vi "RC_STM_Client 1.vi"() -> ()   [LabVIEW 2019, in "RemoteControl.STM.lvclass"]
uses:
  RemoteControl.STM.lvclass
  RemoteControl/RemoteControl.lvclass
  <userlib>/_OpenG.lib/numeric/numeric.llb/Random Number Within Range - I32__ogtk.vi
  <userlib>/_OpenG.lib/error/error.llb/Filter Error Codes (Array)__ogtk.vi
  C:/user/patrick/git/LevyLab-Instrument-Framework/2019 instrument Folder/lvsrc/SMOs/RemoteControl/RemoteControl.lvclass
  C:/user/patrick/git/LevyLab-Instrument-Framework/2019 instrument Folder/lvsrc/SMOs/LevyLab/LevyLab.lvclass
  C:/Program Files (x86)/National Instruments/LabVIEW 2019/vi.lib/JKI/JKI SMO/SMO/SMO.lvclass
panel:
  in  "Test RC Client":bool
  in  "milliseconds to wait":u32
  out "time (1 message) (ms)":u32
  out "startup time (ms)":u32
  out "messsages/s":dbl
  in  "remote port":u16=6341
  in  "address":string
  out "Data reponse":string
  out "Messages":i32
  in  "Stop":bool
  out "Command reponse":string
  out "Command":string
  out "meta data\n(available commands)":string
  out "error out":errorcluster
  # "CLIENT (API)"
  # "Connection info"
  # "Message Sent"
  # "Message Received"
  # "Metrics"
  # "1"
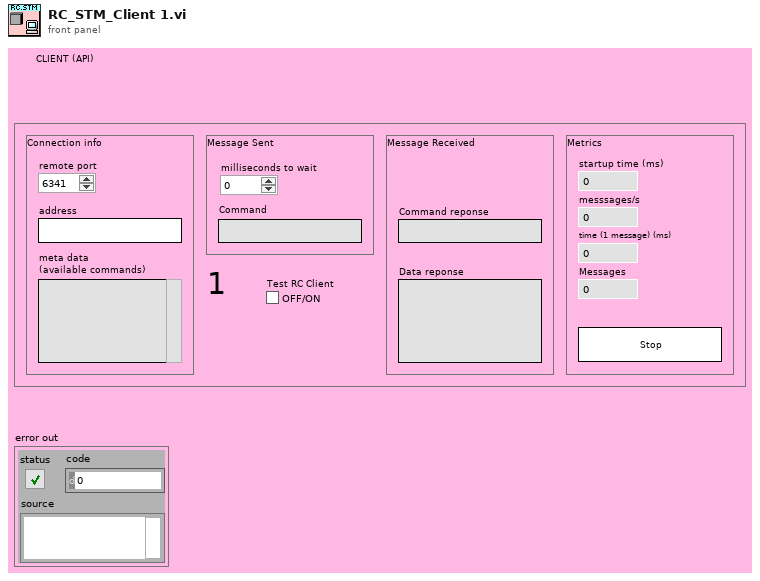
[diagram p1: front panel]
types:
  T1 = typedef "NI STM.lvlib/MetaDataElement.ctl" = string
  T2 = cluster{"Command out":string, "Data out":variant, i32}
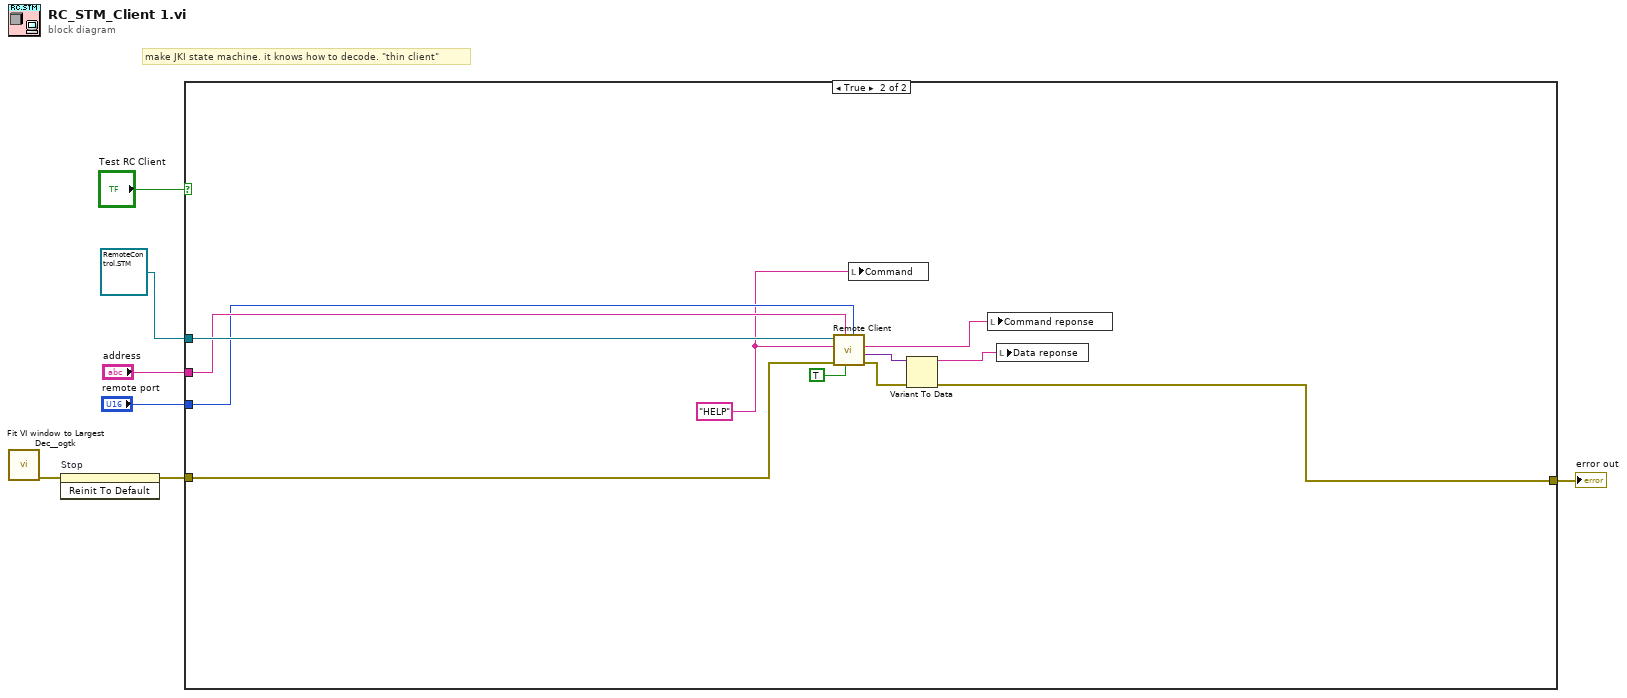
[diagram p0: block diagram]
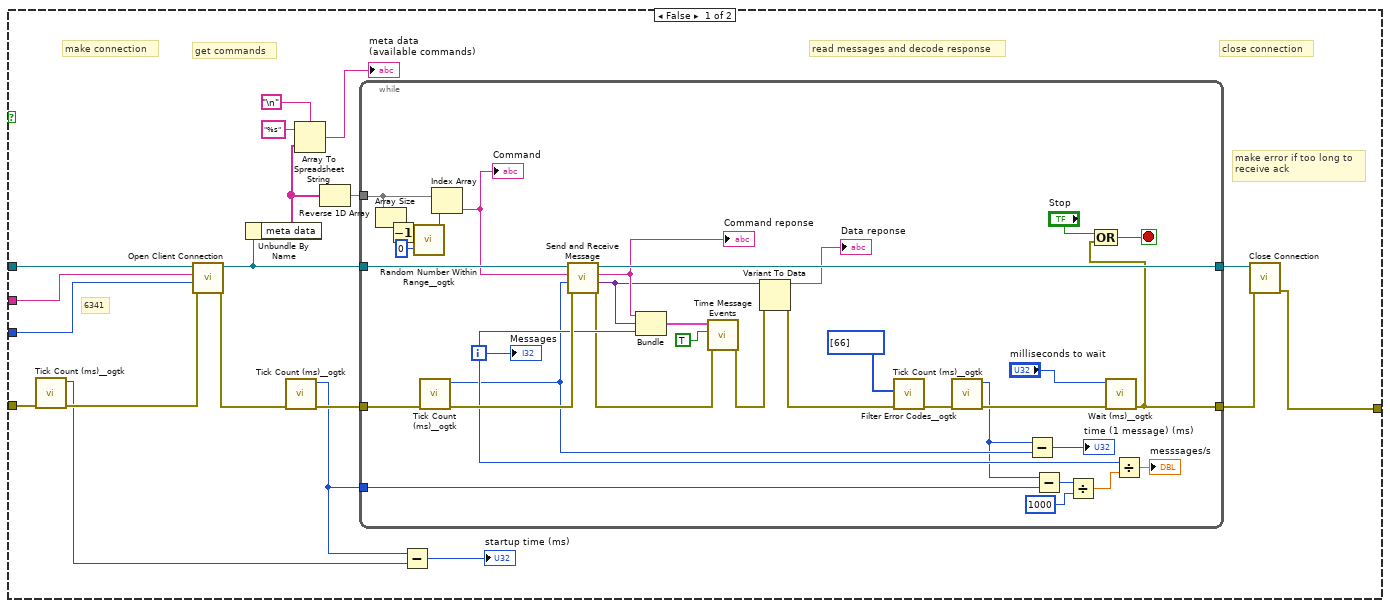
[diagram p2: hidden frame]
diagram:
  # "make JKI state machine. it knows how to decode. \"thin client\""
  n1 = call <userlib>:"Fit VI window to Largest Dec__ogtk.vi"() -> ("error out"=w2:errorcluster)  [unwired: 6 in, 1 out]
  n2 = invoke on="Stop" class="Bool" method="Reinit To Default"(error in=w2) -> (error out=w3:errorcluster)  [unwired: 2 in, 2 out]
  n3 = case shown="True" "Test RC Client" {
    tunnel: refnum<class "RemoteControl.STM.lvclass"> refnum ("RemoteControl.STM in") -> [w12 w71]
    tunnel: "remote port" -> [w11 w63]
    tunnel: "address" -> [w10 w64]
    tunnel: w3 -> [w9 w65]
    tunnel: [w8 w66] -> w1
    frame False {
      # "close connection"
      # "read messages and decode response"
      # "get commands"
      # "make connection"
      # "6341"
      # "make error if too long to\nreceive ack"
      n4 = call <userlib>:"Tick Count (ms)__ogtk.vi"("error in (no error)"=w9) -> ("error out"=w22:errorcluster, "millisecond timer value"=w18:u32)  [unwired: 9 in]
      n5 = call-dynamic "Open Client Connection.vi"("error in (no error)"=w22, "Port"=w11, "address"=w10, "RemoteControl.STM in"=w12) -> ("error out"=w21:errorcluster, "RemoteControl.STM out"=w24:refnum<class "RemoteControl.STM.lvclass">)  [unwired: 6 in]
      n6 = Unbundle By Name(w24) -> ("meta data"=w17:T1[])
      n7 = call <userlib>:"Tick Count (ms)__ogtk.vi"("error in (no error)"=w21) -> ("error out"=w20:errorcluster, "millisecond timer value"=w13:u32)  [unwired: 9 in]
      n8 = Array To Spreadsheet String(delimiter (Tab)="\n", array=w17, 3:"%s" ("format string")) -> (spreadsheet string=→"meta data\n(available commands)":string)
      n9 = Reverse 1D Array(array=w17) -> (reversed array=w23:T1[])
      n10 = while {
        tunnel: [w36] -> w26
        tunnel: [w57] -> w25
        tunnel: w20 -> [w52]
        tunnel: w24 -> [w58]
        tunnel: w23 -> [w40]
        tunnel: w13 -> [w27]
        i -> [w49]
        stop <- w60 stop-if-true
        n11 = Array Size(array=w40) -> (size(s)=w41:i32)
        n12 = Decrement(x=w41) -> (x-1=w39:i32)
        n13 = call-poly <userlib>:"Random Number Within Range__ogtk.vi"("High"=w39, "Low"=0) -> ("Random Number"=w43:i32)  [unwired: 3 in]
        n14 = call <userlib>:"Tick Count (ms)__ogtk.vi"("error in (no error)"=w52) -> ("error out"=w51:errorcluster, "millisecond timer value"=w37:u32)  [unwired: 9 in]
        n15 = Index Array(array=w40, index=w43) -> (element=w53:T1)
        "Command" <- w53
        n16 = call-dynamic "Send and Receive Message.vi"("error in (no error)"=w51, "Data"=w37, "Command"=w53, "RemoteControl in"=w58) -> ("error out"=w38:errorcluster, "Data out"=w35:variant, "Command out"=w50:string, "RemoteControl out"=w57:refnum<class "RemoteControl.STM.lvclass">)  [unwired: 4 in]
        "Command reponse" <- w50
        n17 = Bundle("Command out"=w50, "Data out"=w35, w49) -> (w48:T2)  [unwired: 1 in]
        n18 = call "Time Message Events.vi"("error in (no error)"=w38, "Debug Mode"=TRUE, "Message in"=w48) -> ("error out"=w34:errorcluster)  [unwired: 6 in, 2 out]
        n19 = Variant To Data(error in=w34, Variant=w35) -> (data=→"Data reponse":string, error out=w33:errorcluster)  [unwired: 1 in]
        n20 = call-poly <userlib>:"Filter Error Codes__ogtk.vi"("Error In"=w33, "Error Codes to Filter"=i32[] [66]) -> ("Error Out"=w56:errorcluster)  [unwired: 7 in, 2 out]
        n21 = call <userlib>:"Tick Count (ms)__ogtk.vi"("error in (no error)"=w56) -> ("error out"=w46:errorcluster, "millisecond timer value"=w29:u32)  [unwired: 9 in]
        n22 = Subtract(x=w29, y=w37) -> (x-y=→"time (1 message) (ms)":u32)
        n23 = Subtract(x=w29, y=w27) -> (x-y=w28:u32)
        n24 = Divide(x=w28, y=u32 1000) -> (x/y=w55:dbl)
        n25 = call <userlib>:"Wait (ms)__ogtk.vi"("error in (no error)"=w46, "milliseconds to wait"="milliseconds to wait") -> ("error out"=w36:errorcluster)  [unwired: 8 in, 1 out]
        n26 = Compound Arithmetic op=OR("Stop", w36) -> (w60:bool)
        n27 = Divide(x=w49, y=w55) -> (x/y=→"messsages/s":dbl)
        "Messages" <- w49
      }
      n28 = Subtract(x=w13, y=w18) -> (x-y=→"startup time (ms)":u32)
      n29 = call-dynamic "Close Connection.vi"("error in (no error)"=w26, "RemoteControl.STM in"=w25) -> ("error out"=w8:errorcluster)  [unwired: 8 in, 1 out]
    }
    frame True {
      w62 = "HELP" ("Command")
      n30 = call "Remote Client.vi"("Port"=w63, "Wait for Response?"=TRUE, "address"=w64, "error in (no error)"=w65, "Command"=w62, "RemoteControl in"=w71) -> ("error out"=w67:errorcluster, "Data out"=w70:variant, "Command out"=w69:string)  [unwired: 2 in, 1 out]
      n31 = local write "Command"(w62) -> ()
      n32 = Variant To Data(error in=w67, Variant=w70) -> (data=w68:string, error out=w66:errorcluster)  [unwired: 1 in]
      n33 = local write "Command reponse"(w69) -> ()
      n34 = local write "Data reponse"(w68) -> ()
    }
  }
  "error out" <- w1
